vi "Configure Parameter Conversion.vi"(0 "VISA resource name":refnum<visa-resource-name>, 1 "Channel (1)":i32=1, 3 "Conversion Function State (F: Disable)":bool, 5 "Parameter (0: Z Reflection)":u16(ring) items=["Z Reflection", "Z Transmission", "Y Reflection", "Y Transmission", "Inverse S-parameter", "Z Trans Shunt", "Y Trans Shunt", "Conjugate"], 11 "error in (no error)":errorcluster) -> (4 "VISA resource name out":refnum<visa-resource-name>, 15 "error out":errorcluster)   [LabVIEW 2020, in "Agilent ENA Series.lvlib"]
doc: "Configures the parameter conversion."
uses:
  <instrlib>/Agilent ENA Series/Agilent ENA Series.lvlib
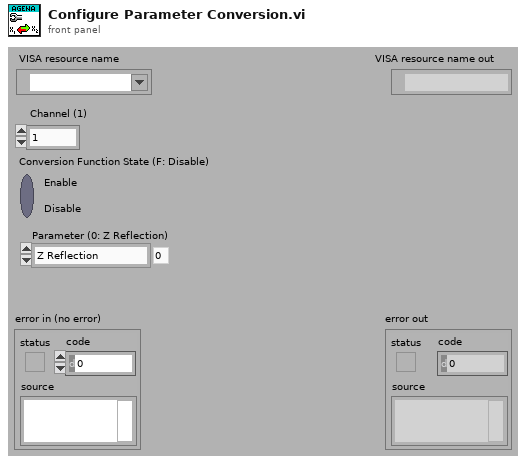
[diagram p1: front panel]
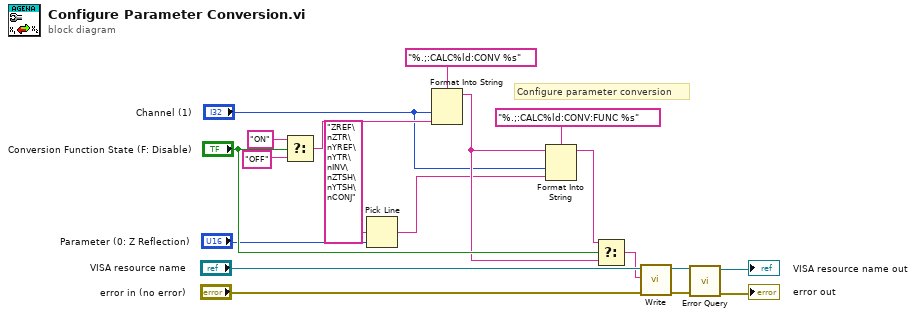
[diagram p0: block diagram]
diagram:
  # "Configure parameter conversion"
  n1 = Select(t="ON", s="Conversion Function State (F: Disable)", f="OFF") -> (s? t:f=w14:string)
  n2 = Pick Line(multi-line string="ZREF\nZTR\nYREF\nYTR\nINV\nZTSH\nYTSH\nCONJ", line index="Parameter (0: Z Reflection)") -> (output string=w8:string)  [unwired: 1 in]
  n3 = Format Into String(format string="%.;:CALC%ld:CONV %s", "Channel (1)", w14) -> (resulting string=w11:string)  [unwired: 2 in, 1 out]
  n4 = Format Into String(format string="%.;:CALC%ld:CONV:FUNC %s", initial string=w11, "Channel (1)", w8) -> (resulting string=w5:string)  [unwired: 1 in, 1 out]
  n5 = Select(t=w5, s="Conversion Function State (F: Disable)", f=w11) -> (s? t:f=w7:string)
  n6 = call <instrlib>:"Write.vi"("error in (no error)"="error in (no error)", "String ()"=w7, "VISA resource name"="VISA resource name") -> ("error out"=w3:errorcluster, "VISA resource name out"=w4:refnum<visa-resource-name>)  [unwired: 6 in, 1 out]
  n7 = call <instrlib>:"Error Query.vi"("error in (no error)"=w3, "VISA resource name"=w4) -> ("error out"=→"error out":errorcluster, "VISA resource name out"=→"VISA resource name out":refnum<visa-resource-name>)  [unwired: 6 in, 2 out]
